vi "Execute.vi"(8 "error in (no error)":errorcluster, 10 "Execution":refnum<data-value>, 11 "UIStepBase in":refnum<class "UIStep.lvclass">) -> (0 "error out":errorcluster, 1 "Output Values":cluster{"Name":string, "Variant Data":variant}[](array[cluster]), 3 "UIStepBase out":refnum<class "UIStep.lvclass">)   [LabVIEW 2015, in "UIStep.lvclass"]
uses:
  UIStep.lvclass
  Execution.lvclass
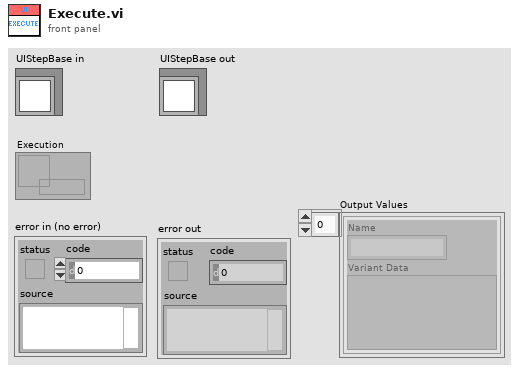
[diagram p1: front panel]
types:
  T1 = cluster{"Embedded":bool, "Size":enum16{"Small", "Middle", "Big"}, "Title":string, "Content":string, "Text Style":cluster{"Font":string, "Size":dbl, "Justification":u16, "TextColor":u32, "BGColor":u32, "Bold":bool}, "Buttons":cluster{"Button1":cluster{"Label":string, "Size":dbl, "TextColor":u32, "BGColor":u32, "Bold":bool}, "Button2":cluster{"Label":string, "Size":dbl, "TextColor":u32, "BGColor":u32, "Bold":bool}}, "Image":path, "Enable Input":bool, "Input Validation":string}
  T2 = cluster{"Font":string, "Size":dbl, "Justification":u16, "TextColor":u32, "BGColor":u32, "Bold":bool}
  T3 = cluster{"Button1":cluster{"Label":string, "Size":dbl, "TextColor":u32, "BGColor":u32, "Bold":bool}, "Button2":cluster{"Label":string, "Size":dbl, "TextColor":u32, "BGColor":u32, "Bold":bool}}
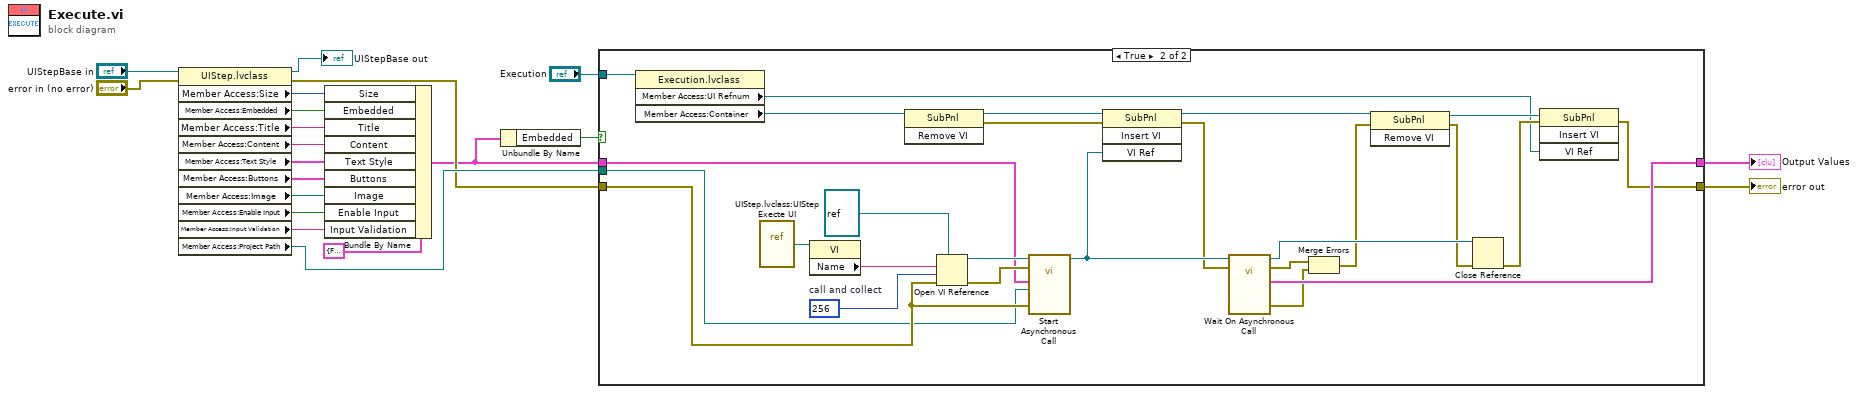
[diagram p0: block diagram]
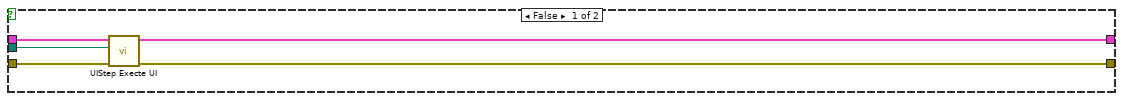
[diagram p2: hidden frame]
diagram:
  n1 = property class="UIStep.lvclass"(reference="UIStepBase in", error in="error in (no error)") -> (reference out=→"UIStepBase out":refnum<class "UIStep.lvclass">, error out=w6:errorcluster, "Member Access:Size"=w4:enum16{"Small", "Middle", "Big"}, "Member Access:Embedded"=w18:bool, "Member Access:Title"=w17:string, "Member Access:Content"=w16:string, "Member Access:Text Style"=w15:T2, "Member Access:Buttons"=w14:T3, "Member Access:Image"=w13:path, "Member Access:Enable Input"=w12:bool, "Member Access:Input Validation"=w11:string, "Member Access:Project Path"=w9:path)
  n2 = Bundle By Name(cluster=T1 {"Embedded"=FALSE, "Size"=enum."Small", "Title"="", "Content"="", "Text Style"={"Font"="", "Size"=0.0, "Justification"=1, "TextColor"=0, "BGColor"=0, "Bold"=FALSE}, "Buttons"={"Button1"={"Label"="", "Size"=0.0, "TextColor"=0, "BGColor"=0, "Bold"=FALSE}, "Button2"={"Label"="", "Size"=0.0, "TextColor"=0, "BGColor"=0, "Bold"=FALSE}}, "Image"=path "", "Enable Input"=FALSE, "Input Validation"=""} ("UI Step Setting"), "Size"=w4, "Embedded"=w18, "Title"=w17, "Content"=w16, "Text Style"=w15, "Buttons"=w14, "Image"=w13, "Enable Input"=w12, "Input Validation"=w11) -> (w3:T1)
  n3 = Unbundle By Name(w3) -> ("Embedded"=w2:bool)
  n4 = case shown="True" w2 {
    tunnel: w9 -> [w25 w43]
    tunnel: [w24 w38] -> w8
    tunnel: w6 -> [w23 w44]
    tunnel: [w22 w28] -> w5
    tunnel: w3 -> [w21 w42]
    tunnel: "Execution" -> [_ w51]
    frame False {
      n5 = call "UIStep Execte UI.vi"("error in (no error)"=w23, "Project Path"=w25, "UI Setting"=w21) -> ("error out"=w22:errorcluster, "Output Values"=w24:cluster{"Name":string, "Variant Data":variant}[])  [unwired: 7 in]
    }
    frame True {
      w48 = 256  # call and collect
      n6 = property class="Execution.lvclass"(reference=w51) -> ("Member Access:UI Refnum"=w26:refnum<vi>, "Member Access:Container"=w27:refnum<vi>)  [unwired: 1 in, 2 out]
      n7 = vi-ref "UIStep.lvclass:UIStep Execte UI.vi"() -> (w50:refnum<vi>)
      n8 = property class="VI"(reference=w50) -> ("Name"=w49:string)  [unwired: 1 in, 2 out]
      n9 = invoke class="SubPnl" method="Remove VI"(reference=w27) -> (reference out=w41:refnum<vi>, error out=w30:errorcluster)  [unwired: 2 in, 1 out]
      n10 = Open VI Reference(type specifier VI Refnum (for type only)=refnum<vi> refnum, vi path=w49, options=w48, error in (no error)=w44) -> (vi reference=w46:refnum<vi>, error out=w45:errorcluster)  [unwired: 2 in]
      n11 = call-by-ref "Start Asynchronous Call"(reference=w46, error in=w45, 8:"error in (no error)"=w44, "Project Path"=w43, "UI Setting"=w42) -> (reference out=w40:refnum<vi>)  [unwired: 7 in, 3 out]
      n12 = invoke class="SubPnl" method="Insert VI"(reference=w41, error in=w30, "VI Ref"=w40) -> (reference out=w34:refnum<vi>, error out=w39:errorcluster)  [unwired: 1 in, 2 out]
      n13 = call-by-ref "Wait On Asynchronous Call"(reference=w40, error in=w39) -> (reference out=w37:refnum<vi>, error out=w36:errorcluster, 0:"error out"=w35:errorcluster, "Output Values"=w38:cluster{"Name":string, "Variant Data":variant}[])  [unwired: 10 in]
      n14 = Merge Errors(w36, w35) -> (w32:errorcluster)
      n15 = invoke class="SubPnl" method="Remove VI"(reference=w34, error in=w32) -> (reference out=w33:refnum<vi>, error out=w31:errorcluster)  [unwired: 1 in, 1 out]
      n16 = Close Reference(reference=w37, error in (no error)=w31) -> (error out=w29:errorcluster)
      n17 = invoke class="SubPnl" method="Insert VI"(reference=w33, error in=w29, "VI Ref"=w26) -> (error out=w28:errorcluster)  [unwired: 1 in, 3 out]
    }
  }
  "error out" <- w5
  "Output Values" <- w8
